vi "RSZVB Calibration Auto Assignment Type.vi"(7 "Calibration Kit Name (\"\")":string, 8 "error in (no error)":errorcluster {"code" format="%.0x"}, 9 "Parameters (Full N-port)":i32(ring)=10 items=["Full One Port"=2, "One Path Two Port"=4, "Full N-port"=10], 10 "Channel (1)":i32=1, 11 "VISA resource name":refnum<visa-resource-name>) -> (0 "error out":errorcluster {"code" format="%.0x"}, 3 "VISA resource name out":refnum<visa-resource-name>)   [LabVIEW 2011]
doc: "This VI selects a calibration type and a cal unit characterization (cal kit file) for an automatic calibration with multiple port assignments. \n\nRemote-control command(s):\n[SENSe<Ch>:]CORRection:COLLect:AUTO:CONFigure <cal_type>, '<file_name>'}"
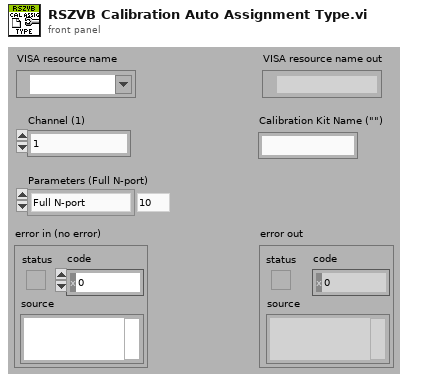
[diagram p1: front panel]
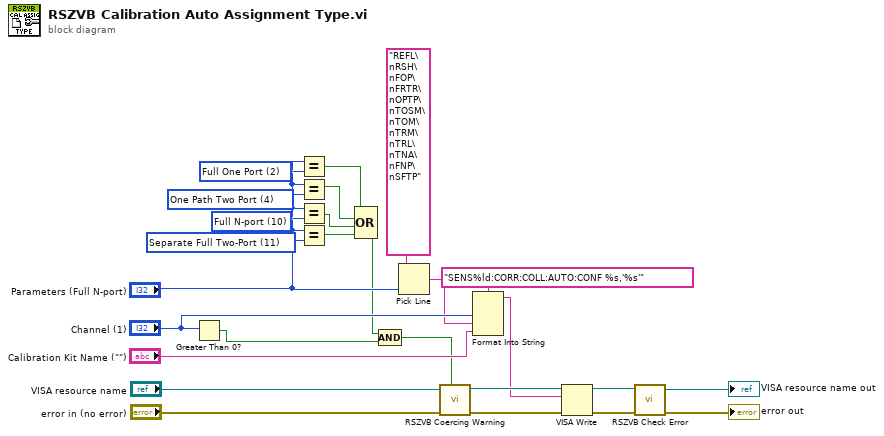
[diagram p0: block diagram]
diagram:
  w12 = 11 items=["Full One Port"=2, "One Path Two Port"=4, "Full N-port"=10, "Separate Full Two-Port"=11] ("Parameters (2: Full One Port)")
  w19 = 10 items=["Full One Port"=2, "One Path Two Port"=4, "Full N-port"=10, "Separate Full Two-Port"=11] ("Parameters (2: Full One Port)")
  w18 = 4 items=["Full One Port"=2, "One Path Two Port"=4, "Full N-port"=10, "Separate Full Two-Port"=11] ("Parameters (2: Full One Port)")
  w17 = 2 items=["Full One Port"=2, "One Path Two Port"=4, "Full N-port"=10, "Separate Full Two-Port"=11] ("Parameters (2: Full One Port)")
  n1 = Greater Than 0?(x="Channel (1)") -> (x > 0?=w7:bool)
  n2 = Equal?(x="Parameters (Full N-port)", y=w17) -> (x = y?=w16:bool)
  n3 = Equal?(x="Parameters (Full N-port)", y=w18) -> (x = y?=w15:bool)
  n4 = Equal?(x="Parameters (Full N-port)", y=w19) -> (x = y?=w14:bool)
  n5 = Equal?(x="Parameters (Full N-port)", y=w12) -> (x = y?=w13:bool)
  n6 = Compound Arithmetic op=OR(w16, w15, w14, w13) -> (w8:bool)
  n7 = Compound Arithmetic op=AND(w8, w7) -> (w4:bool)
  n8 = Pick Line(multi-line string="REFL\nRSH\nFOP\nFRTR\nOPTP\nTOSM\nTOM\nTRM\nTRL\nTNA\nFNP\nSFTP", line index="Parameters (Full N-port)") -> (output string=w6:string)  [unwired: 1 in]
  n9 = call "RSZVB Coercing Warning.vi"("In Range?"=w4, "error in (no error)"="error in (no error)", "VISA session"="VISA resource name") -> ("error out"=w26:errorcluster, "dup VISA session"=w25:refnum<visa-resource-name>)  [unwired: 7 in]
  n10 = Format Into String(format string="SENS%ld:CORR:COLL:AUTO:CONF %s,'%s'", "Channel (1)", w6, "Calibration Kit Name (\"\")") -> (resulting string=w3:string)  [unwired: 2 in, 1 out]
  n11 = VISA Write(VISA resource name=w25, write buffer=w3, error in (no error)=w26) -> (VISA resource name out=w23:refnum<visa-resource-name>, error out=w24:errorcluster)  [unwired: 1 out]
  n12 = call "RSZVB Check Error.vi"("error in (no error)"=w24, "VISA session"=w23) -> ("error out"=→"error out":errorcluster, "dup VISA session"=→"VISA resource name out":refnum<visa-resource-name>)  [unwired: 8 in]
